vi "Fail With Popup.vi"(1 "String":string) -> ()   [LabVIEW 2013]
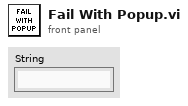
[diagram p1: front panel]
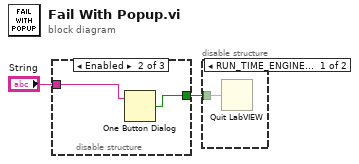
[diagram p0: block diagram]
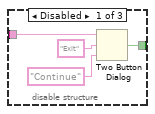
[diagram p2: hidden frame]
diagram:
  n1 = disable-structure shown="Enabled" {
    disable-tunnel: "String" -> [w6 w8 _]
    disable-tunnel: [w3 w7 _] -> w1
    frame Disabled {
      n2 = Two Button Dialog(message=w6, 1:"Continue" ("F button name (\"Cancel\")"), 2:"Exit" ("T button name (\"OK\")")) -> (T button?=w3:bool)
    }
    frame Enabled {
      n3 = One Button Dialog(message=w8) -> (true=w7:bool)  [unwired: 1 in]
    }
    frame Disabled {
    }
  }
  n4 = disable-structure shown="RUN_TIME_ENGINE==True" {
    disable-tunnel: w1 -> [w9 _]
    frame condition #0 {
      n5 = Quit LabVIEW(quit? (T)=w9) -> ()
    }
    frame condition #1 (active) {
    }
  }
